vi "Simplify VI Name.vi"(11 "Full Qualified Name":string) -> (3 "Simple Name":string)   [LabVIEW 2020, in "Peek Window.lvlib"]
uses:
  Peek Window.lvlib
  <vilib>/regexp/Match Regular Expression.xnode
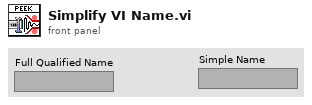
[diagram p1: front panel]
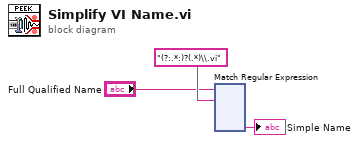
[diagram p0: block diagram]
diagram:
  n1 = xnode "Match Regular Expression"("input string"="Full Qualified Name", "regular expression"="(?:.*:)?(.*)\\.vi") -> ("submatch 1"=→"Simple Name":string)  [unwired: 4 in, 5 out]
